vi "Pre Launch Init.vi"(11 "IEventAggregator in":refnum<class "IEventAggregator.lvclass">) -> (0 "error out":errorcluster, 3 "IEventAggregator out":refnum<class "IEventAggregator.lvclass">)   [LabVIEW 2015, in "ActorEvents.lvlib" / "IEventAggregator.lvclass"]
doc: "(<B>Filename</B>: Actor Framework.lvlib:Actor.lvclass:Pre Launch Init.vi)\n\nDefines behavior that occurs after the Launch Nested Actor method is invoked but before the actor's Actor Core method begins running.\n\nBy default, this method does nothing. A descendant class may override it to define behavior."
uses:
  IEventAggregator.lvclass
  <vilib>/ActorFramework/Actor/Actor.lvclass/Actor.ctl
  <vilib>/ActorFramework/Message Enqueuer/Message Enqueuer.lvclass/Message Enqueuer.ctl
  <vilib>/ActorFramework/Message Enqueuer/Init from Existing Queue.vi
  <vilib>/ActorFramework/Message Enqueuer/Enqueue.vi
  <vilib>/ActorFramework/Message Priority Queue/Priority Enqueue.vi
  IObserver/IObserver/IObserver.lvclass
  AutoEventActor Messages/Launch Event Handlers Msg/Launch Event Handlers Msg.lvclass
  <vilib>/ActorFramework/Message Enqueuer/Message Enqueuer.lvclass
  <vilib>/ActorFramework/Actor/Actor.lvclass
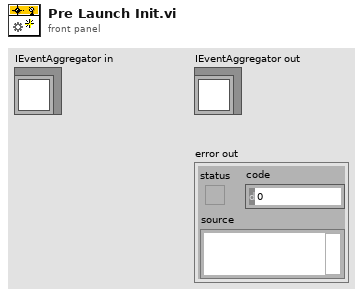
[diagram p1: front panel]
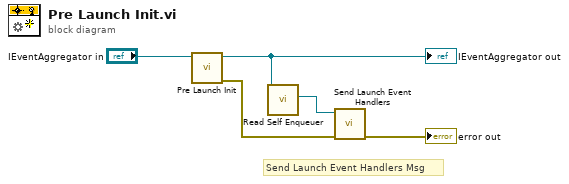
[diagram p0: block diagram]
diagram:
  # "Send Launch Event Handlers Msg"
  n1 = call-parent "Pre Launch Init.vi"("Actor in"="IEventAggregator in") -> ("error out"=w4:errorcluster, "Actor out"=w2:refnum<class "IEventAggregator.lvclass">)  [unwired: 9 in]
  "IEventAggregator out" <- w2
  n2 = call <vilib>:"Read Self Enqueuer.vi"("Actor"=w2) -> ("Self Enqueuer"=w1:refnum<class "Message Enqueuer.lvclass">)  [unwired: 10 in]
  n3 = call "Send Launch Event Handlers.vi"("error in (no error)"=w4, "Message Enqueuer (EventAggregator)"=w1) -> ("error out"=→"error out":errorcluster)  [unwired: 8 in, 1 out]
